vi "FTW-Socket-Core-ReturnCode.vi"(0 "error in":errorcluster, 7 "Return Code":i64) -> (4 "error out":errorcluster)   [LabVIEW 2015]
panel:
  # "Inputs"
  # "Outputs"
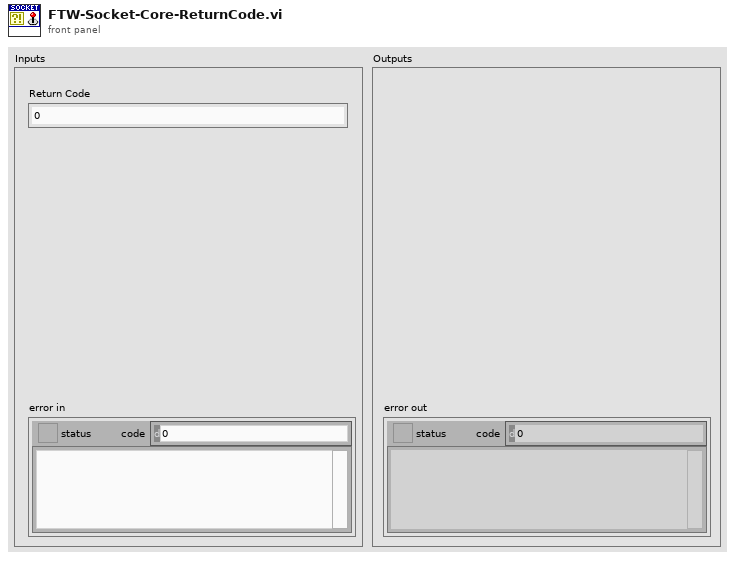
[diagram p1: front panel]
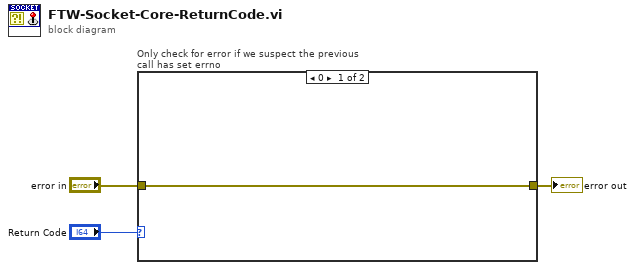
[diagram p0: block diagram]
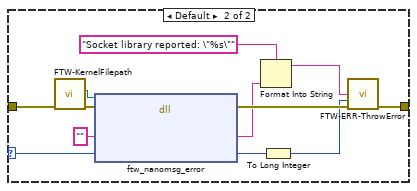
[diagram p2: hidden frame]
diagram:
  n1 = case "Only check for error if we suspect the previous call has set errno" shown="0" "Return Code" {
    selector: "Return Code" -> [_ w10]
    tunnel: [w4 w16] -> w3
    tunnel: "error in" -> [w4 w13]
    frame 0 {
    }
    frame Default {
      n2 = call "FTW-KernelFilepath.vi"("error in"=w13) -> ("error out"=w12:errorcluster, "Library Filepath"=w11:path)  [unwired: 8 in, 1 out]
      n3 = dll-call lib="?" fn="ftw_nanomsg_error"(path in=w11, error in=w12, "Message"="", "Return Code"=w10) -> (error out=w15:errorcluster, "Message"=w7:string, "Return Code"=w6:i64)  [unwired: 2 in, 1 out]
      n4 = Format Into String(format string="Socket library reported: \"%s\"" ("Error Message"), w7) -> (resulting string=w8:string)  [unwired: 2 in, 1 out]
      n5 = To Long Integer(number=w6) -> (32bit integer=w5:i32)
      n6 = call "FTW-ERR-ThrowError.vi"("Error Message"=w8, "Error Code"=w5, "error in"=w15) -> ("error out"=w16:errorcluster)  [unwired: 12 in]
    }
  }
  "error out" <- w3
